vi "Acc Limit.vi"(8 "Trans De-Acc":dbl, 9 "Trans Acc":dbl, 10 "Past Setpoint":cluster{"x":dbl, "y":dbl}, 11 "Current Setpoint":cluster{"x":dbl, "y":dbl}) -> (3 "Trans Vel out":cluster{"x":dbl, "y":dbl})   [LabVIEW 2020]
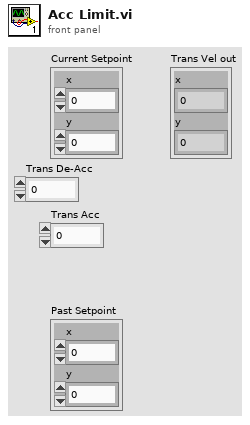
[diagram p1: front panel]
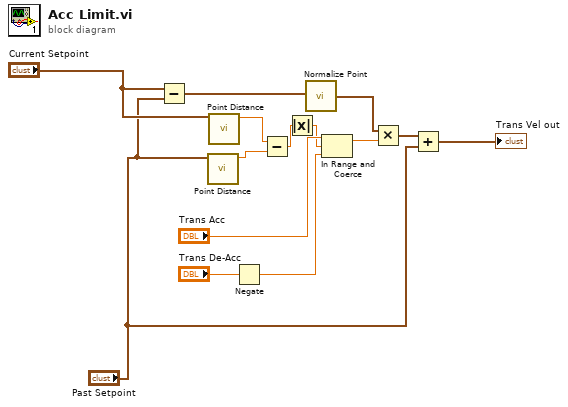
[diagram p0: block diagram]
diagram:
  n1 = Subtract(x="Current Setpoint", y="Past Setpoint") -> (x-y=w9:cluster{"x":dbl, "y":dbl})
  n2 = call "Point Distance.vi"("point a"="Past Setpoint") -> ("dist"=w12:sgl)  [unwired: 10 in]
  n3 = call "Point Distance.vi"("point a"="Current Setpoint") -> ("dist"=w13:sgl)  [unwired: 10 in]
  n4 = Negate(x="Trans De-Acc") -> (-x=w4:dbl)
  n5 = Subtract(x=w13, y=w12) -> (x-y=w2:sgl)
  n6 = Absolute Value(x=w2) -> (abs(x)=w1:sgl)
  n7 = call "Normalize Point.vi"("point in"=w9) -> ("point out"=w8:cluster{"x":sgl, "y":sgl})
  n8 = In Range and Coerce(upper limit="Trans Acc", x=w1, lower limit=w4) -> (coerced(x)=w10:dbl)  [unwired: 1 out]
  n9 = Multiply(x=w8, y=w10) -> (x*y=w7:cluster{"x":dbl, "y":dbl})
  n10 = Add(x=w7, y="Past Setpoint") -> (x+y=→"Trans Vel out":cluster{"x":dbl, "y":dbl})
